vi "Render.vi"(7 "Renderer":refnum<class "Renderer.lvclass">, 8 "error in (no error)":errorcluster, 10 "Camera":refnum<class "Camera.lvclass">, 11 "Element in":refnum<class "Element.lvclass">) -> (0 "error out":errorcluster)   [LabVIEW 2021, in "Element.lvclass"]
uses:
  Element.lvclass
  Camera/Camera.lvclass
  Renderer/Renderer.lvclass
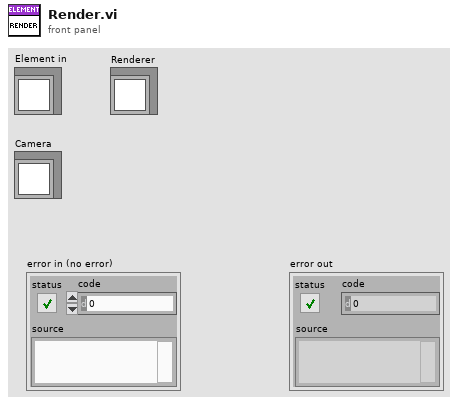
[diagram p1: front panel]
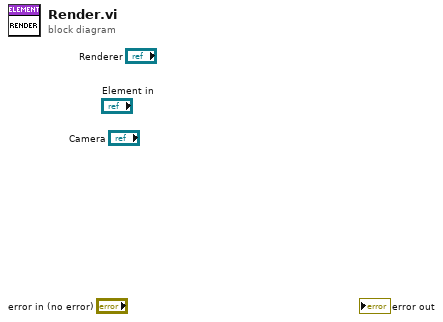
[diagram p0: block diagram]
diagram:
